vi "Buzzer (SubVI).vi"(8 "error in (no error)":errorcluster, 9 "Buzzer's channel":i32, 10 "LINX Resource":T1, 11 "Melody (frequency:duration)":dbl[][](array[numeric])) -> ()   [LabVIEW 2014]
uses:
  <vilib>/MakerHub/LINX/Private/Type Defs/LINX Ref.ctl
  <vilib>/MakerHub/LINX/Private/Type Defs/Platform.ctl
  <vilib>/MakerHub/LINX/Private/Type Defs/Interface.ctl
  <vilib>/MakerHub/LINX/Private/Device/Type Defs/LINX Device Config.ctl
  <vilib>/MakerHub/LINX/Private/Device/Type Defs/TCP Config.ctl
  <vilib>/MakerHub/LINX/Private/Device/Type Defs/Channels.ctl
  <vilib>/MakerHub/LINX/Public/Peripherals/Digital/Digital Write 1 Chan.vi
  <vilib>/MakerHub/LINX/Public/Peripherals/Digital/Digital Write N Chans.vi
  <vilib>/MakerHub/LINX/Private/Local IO/LinxDigitalWrite.vi
  <vilib>/MakerHub/LINX/Public/Utilities/Check Channel.vi
  <vilib>/MakerHub/LINX/Private/Local IO/Handle Errors.vi
  <vilib>/MakerHub/LINX/Private/Utilties/Generate Error.vi
  <vilib>/MakerHub/LINX/LMH-LINX.lvlib
  <vilib>/MakerHub/LINX/Private/Device/Device.lvlib
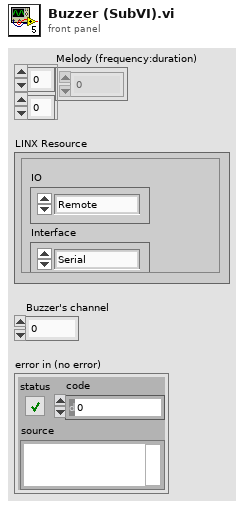
[diagram p1: front panel]
types:
  T1 = typedef "LMH-LINX.lvlib/LINX Ref.ctl" = cluster{"IO":T2, "Interface":T3, "LINX Device Config":T4}
  T2 = typedef "LMH-LINX.lvlib/Platform.ctl" = enum16{"Remote", "Local"}
  T3 = typedef "LMH-LINX.lvlib/Interface.ctl" = enum16{"Serial", "TCP"}
  T4 = typedef "LMH-LINX.lvlib/Device.lvlib/LINX Device Config.ctl" = cluster{"Interface":T3, "COM Port":refnum<visa-resource-name>, "TCP Configuration":T5, "Device Family":u8, "Device ID":u8, "Device Name":string, "TCP Ref":refnum<k5>, "Channels":T6}
  T5 = typedef "LMH-LINX.lvlib/Device.lvlib/TCP Config.ctl" = cluster{"IP Address":string, "Port":u16}
  T6 = typedef "LMH-LINX.lvlib/Channels.ctl" = cluster{"DI":u8[], "DO":u8[], "AI":u8[], "AO":u8[], "PWM":u8[], "QE":u8[], "UART":u8[], "I2C 2":u8[], "SPI":u8[], "CAN":u8[], "Servo":u8[], "AI Ref (V)":dbl, "AI Resolution (Bits)":u8, "AO Ref (V)":dbl, "AO Resolution (Bits)":u8}
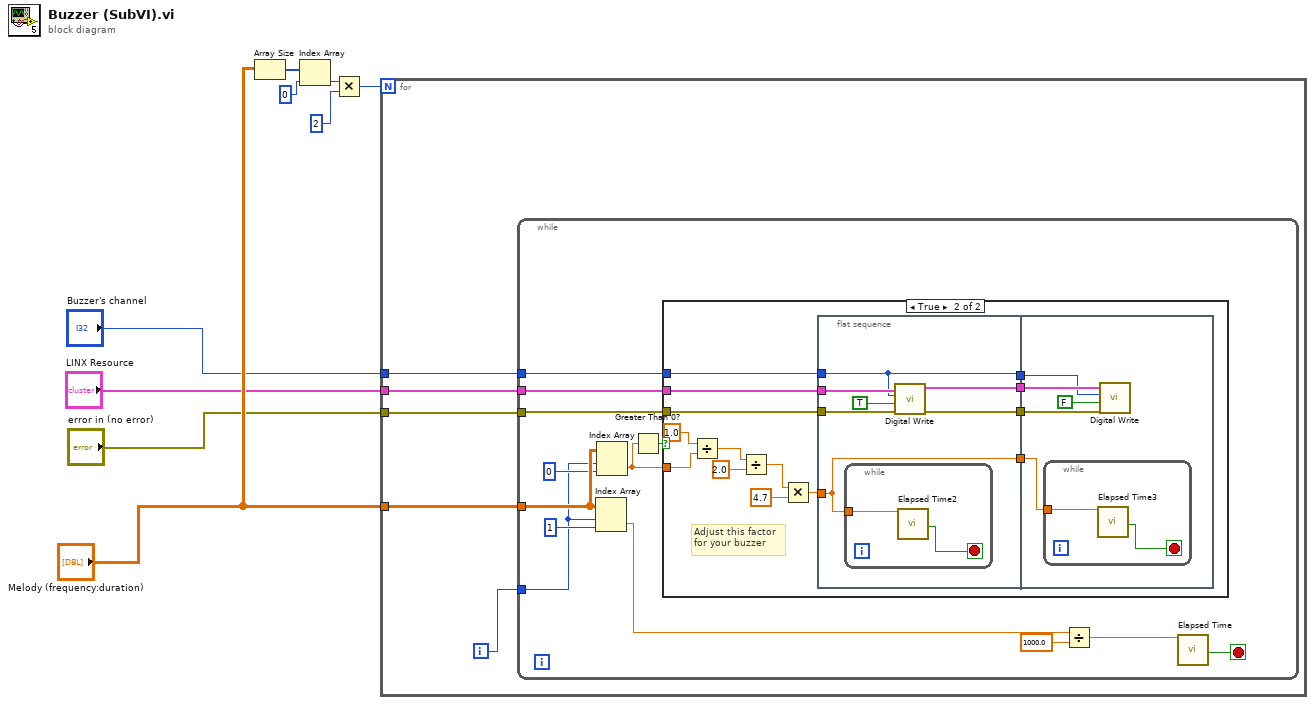
[diagram p0: block diagram]
diagram:
  n1 = Array Size(array="Melody (frequency:duration)") -> (size(s)=w5:i32[])
  n2 = Index Array(array=w5, index=0) -> (element=w6:i32)
  n3 = Multiply(x=w6, y=2) -> (x*y=w8:i32)
  n4 = for {
    N: w8 -> [_]
    tunnel: "LINX Resource" -> [w14]
    tunnel: "error in (no error)" -> [w13]
    tunnel: "Melody (frequency:duration)" -> [w11]
    tunnel: "Buzzer's channel" -> [w12]
    i -> [w10]
    n5 = while {
      tunnel: w14 -> [w27]
      tunnel: w13 -> [w26]
      tunnel: w11 -> [w23]
      tunnel: w10 -> [w20]
      tunnel: w12 -> [w19]
      stop <- w25 stop-if-true
      n6 = Index Array(array=w23, index (row)=w20, index (col)=1 ("disabled index (col)")) -> (element=w17:dbl)
      n7 = Index Array(array=w23, index (row)=w20, index (col)=0 ("disabled index (col)")) -> (element=w15:dbl)
      n8 = Greater Than 0?(x=w15) -> (x > 0?=w16:bool)
      n9 = case shown="True" w16 {
        tunnel: w27 -> [_ w37]
        tunnel: w26 -> [_ w36]
        tunnel: w15 -> [_ w28]
        tunnel: w19 -> [_ w32]
        frame False {
        }
        frame True {
          # "Adjust this factor\nfor your buzzer"
          n10 = Divide(x=1.0, y=w28) -> (x/y=w33:dbl)
          n11 = Divide(x=w33, y=2.0) -> (x/y=w31:dbl)
          n12 = Multiply(x=w31, y=4.7) -> (x*y=w30:dbl)
          n13 = flat-sequence {
            tunnel: w37 -> [w47]
            tunnel: [w46] -> w41
            tunnel: w32 -> [w45]
            tunnel: [w45] -> w40
            tunnel: w36 -> [w44]
            tunnel: [w43] -> w39
            tunnel: w30 -> [w42]
            tunnel: [w42] -> w38
            tunnel: w41 -> [w54]
            tunnel: w40 -> [w53]
            tunnel: w39 -> [w52]
            tunnel: w38 -> [w51]
            frame #0 {
              n14 = while {
                tunnel: w42 -> [w49]
                stop <- w50 stop-if-true
                n15 = call "Elapsed Time2"("Time Target (s)"=w49) -> ("Time has Elapsed"=w50:bool)  [unwired: 11 in, 7 out]
              }
              n16 = call-poly <vilib>:"Digital Write.vi"("Error In"=w44, "Output Value"=TRUE, "DO Channel"=w45, "LINX Resource"=w47) -> ("Error Out"=w43:errorcluster, "LINX Resource"=w46:T1)  [unwired: 6 in]
            }
            frame #1 {
              n17 = while {
                tunnel: w51 -> [w56]
                stop <- w57 stop-if-true
                n18 = call "Elapsed Time3"("Time Target (s)"=w56) -> ("Time has Elapsed"=w57:bool)  [unwired: 11 in, 7 out]
              }
              n19 = call-poly <vilib>:"Digital Write.vi"("Error In"=w52, "Output Value"=FALSE, "DO Channel"=w53, "LINX Resource"=w54) -> ()  [unwired: 6 in, 2 out]
            }
          }
        }
      }
      n20 = Divide(x=w17, y=1000.0) -> (x/y=w18:dbl)
      n21 = call "Elapsed Time"("Time Target (s)"=w18) -> ("Time has Elapsed"=w25:bool)  [unwired: 11 in, 7 out]
    }
  }
